vi "Main Loop.vi"(8 "error in (no error)":errorcluster, 11 "Queue in":refnum<queue>) -> (0 "error out":errorcluster)   [LabVIEW 2015, in "Logger.lvlib"]
uses:
  Logger.lvlib
  support/Message Queue/Message Queue.lvlib
  TypeDefs/Logger State.ctl
  TypeDefs/Logger Data.ctl
  PL Model/API/Get Model Status Control.ctl
  PL Model/PL Model.lvlib
  support/Message Queue/Message Cluster.ctl
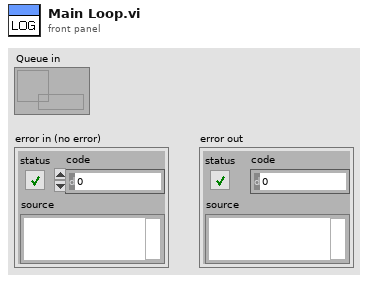
[diagram p1: front panel]
types:
  T1 = typedef "Logger.lvlib/Logger Data.ctl" = cluster{"tdms file out":refnum<k34>, "State":T2}
  T2 = typedef "Logger.lvlib/Logger State.ctl" = enum16{"Idle", "Working"}
  T3 = typedef "PL Model.lvlib/Get Model Status Control.ctl" = cluster{"Position":dbl, "Pump State":bool, "Fluid Flow":dbl, "Fluid Level":dbl, "Barrel Number":i32, "Spill Alarm":bool, "Level Alarm":bool}
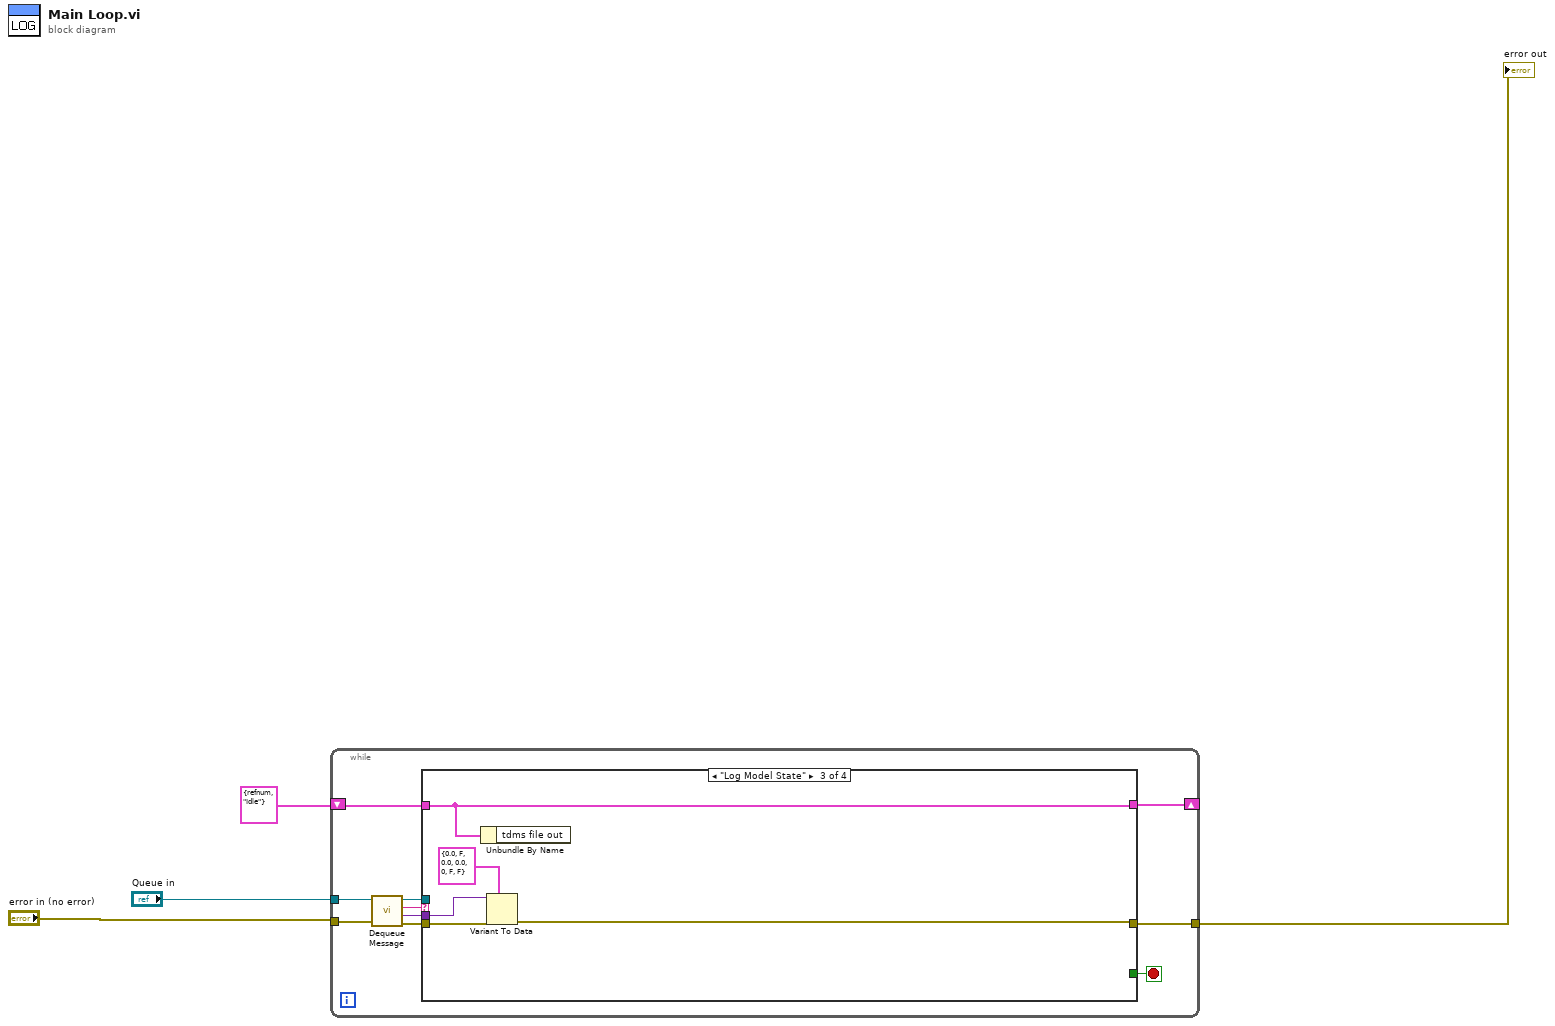
[diagram p0: block diagram]
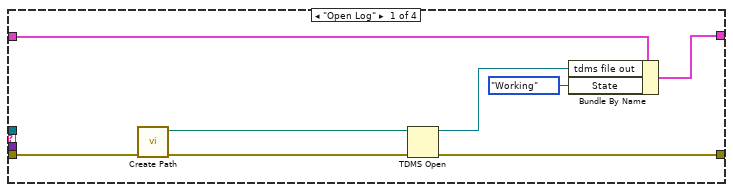
[diagram p2: hidden frame]
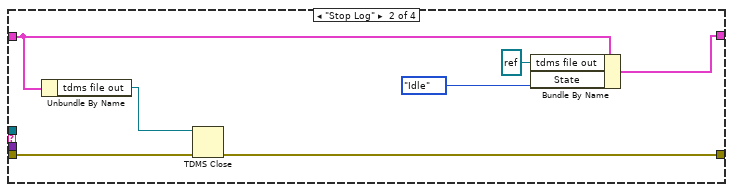
[diagram p3: hidden frame]
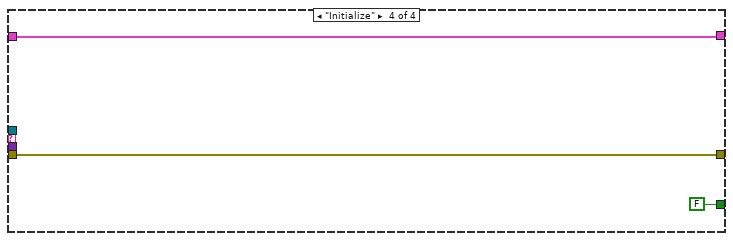
[diagram p4: hidden frame]
diagram:
  n1 = while {
    tunnel: "error in (no error)" -> [w14]
    tunnel: "Queue in" -> [w13]
    tunnel: [w8] -> w2
    shift-right: [w5] -> _
    shift-left: T1 {"tdms file out"=refnum, "State"=enum."Idle"} -> [w6]
    stop <- w7 stop-if-true
    n2 = call "Dequeue Message.vi"("error in (no error)"=w14, "Message Queue"=w13) -> ("error out"=w12:errorcluster, "Message Data"=w9:variant, "Message"=w11:string, "dup Message Queue"=w10:refnum<queue>)  [unwired: 6 in]
    n3 = case shown="\"Log Model State\"" w11 {
      tunnel: w12 -> [w18 w29 w33 w37]
      tunnel: w10 -> [_ _ _ _]
      tunnel: w9 -> [_ _ w31 _]
      tunnel: [w22 w27 w30 w37] -> w8
      tunnel: [_ _ _ FALSE] -> w7
      tunnel: w6 -> [w21 w26 w34 w35]
      tunnel: [w19 w25 w34 w35] -> w5
      frame "Open Log" {
        n4 = call "Create Path.vi"("error in (no error)"=w18) -> ("error out"=w17:errorcluster, "File Path Control"=w16:path)  [unwired: 9 in]
        n5 = TDMS Open(8:w17, 11:w16) -> (0:w22:errorcluster, 3:w20:refnum<k34>)  [unwired: 5 in]
        n6 = Bundle By Name(cluster=w21, "tdms file out"=w20, "State"=Logger_State."Working") -> (w19:T1)
      }
      frame "Stop Log" {
        n7 = Unbundle By Name(w26) -> ("tdms file out"=w28:refnum<k34>)
        n8 = TDMS Close(8:w29, 11:w28) -> (0:w27:errorcluster)  [unwired: 1 out]
        n9 = Bundle By Name(cluster=w26, "tdms file out"=refnum<k34> refnum, "State"=Logger_State."Idle") -> (w25:T1)
      }
      frame "Log Model State" {
        n10 = Unbundle By Name(w34) -> ()  [unwired: 1 out]
        n11 = Variant To Data(error in=w33, type=T3 {"Position"=0.0, "Pump State"=FALSE, "Fluid Flow"=0.0, "Fluid Level"=0.0, "Barrel Number"=0, "Spill Alarm"=FALSE, "Level Alarm"=FALSE} ("Model Status"), Variant=w31) -> (error out=w30:errorcluster)  [unwired: 1 out]
      }
      frame "Initialize" {
      }
    }
  }
  "error out" <- w2
